vi "Drive Controller.vi"(8 "error in":errorcluster) -> ()   [LabVIEW 2019]
doc: "This VI executes continuously carrying out the current operation and responding to updates or new operation requests. It will often contain the timing or control code that is difficult to place directly in TeleOp. This VI generally opens all sensors and motors and isolates the rest of the robot code from knowing implementation details of how the operations are carried out."
uses:
  <vilib>/Rock Robotics/WPI/Framework/Completion Status.ctl
  Drive Setpoints.ctl
  Drive Operations.ctl
  <vilib>/Rock Robotics/WPI/ThirdParty/REV Robotics/SPARK MAX/Typedef/Spark MAX Control Type.ctl
panel:
  in  "Interactive Values":T1
  in  "Buttons":cluster{"Execute Cmd":bool, "Abort Cmd":bool}
  out "Command Timing":cluster{"Start Time (ms)":u32, "Iterations":i32}
  out "Status":T3
  out "Current\nCmd":string
  # "Tip: The graph shows the motor setpoints. It may also be helpful to observe inputs and sensor values.\nYou may also want to display tuning or debugging controls."
  # "Interactive Command: You may fill in the settings for a command\nand schedule it with the Execute button. You can observe and abort\nany command while fine tuning the code for the controller."
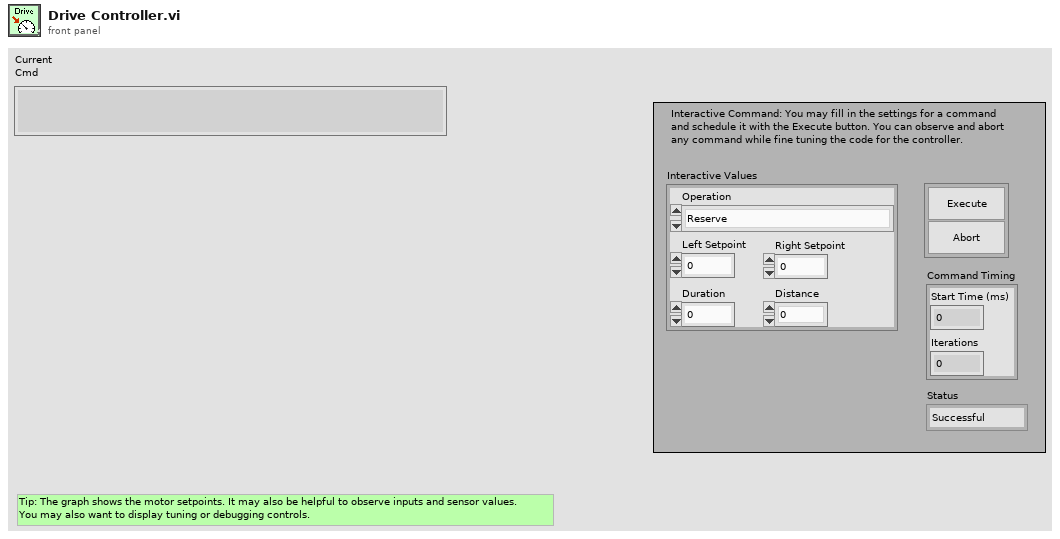
[diagram p1: front panel]
types:
  T1 = typedef "Drive Setpoints.ctl" = cluster{"Operation":T2, "Left Setpoint":dbl, "Right Setpoint":dbl, "Duration":dbl, "Distance":dbl}
  T2 = typedef "Drive Operations.ctl" = enum16{"Reserve", "Read Current", "Immediate", "Drive for Time", "Drive for Distance"}
  T3 = typedef "Completion Status.ctl" = enum16{"Successful", "Aborted", "Incomplete"}
  T4 = typedef "WPI_MotorControlDeviceRef.ctl" = cluster{"DeviceStatus":errorcluster, "Type":T5, "PWM":cluster{"PWM Channel":T6, "DeadBand":T7}, "CAN":cluster{"Device Number":u8, "SetOutput VI Ref":variant, "GetOutput VI Ref":variant, "Enable VI Ref":variant, "Disable VI Ref":variant, "Data":variant}, "Invert":bool, "DIO PWM":cluster{"PWM \"Enable\" Channel":T6, "DIOChannel":T8, "PWM Rate":dbl}}
  T5 = typedef "WPI_MotorControlType.ctl" = enum16{"PWM", "CAN", "DIO PWM"}
  T6 = typedef "FPGA_DIOPWMChannel.ctl" = enum8{"PWM 0", "PWM 1", "PWM 2", "PWM 3", "PWM 4", "PWM 5", "PWM 6", "PWM 7", "PWM 8", "PWM 9", "PWM MXP 0", "PWM MXP 1", "PWM MXP 2", "PWM MXP 3", "PWM MXP 4", "PWM MXP 5", "PWM MXP 6", "PWM MXP 7", "PWM MXP 8", "PWM MXP 9", "Invalid"}
  T7 = typedef "WPI_PWMDeadband.ctl" = cluster{"Name":string, "maxPositivePwm":i32, "minPositivePwm":i32, "centerPwm":i32, "maxNegativePwm":i32, "minNegativePwm":i32, "angularRange":u16}
  T8 = typedef "FPGA_DIOChannel.ctl" = enum8{"DIO 0", "DIO 1", "DIO 2", "DIO 3", "DIO 4", "DIO 5", "DIO 6", "DIO 7", "DIO 8", "DIO 9", "DIO MXP 0", "DIO MXP 1", "DIO MXP 2", "DIO MXP 3", "DIO MXP 4", "DIO MXP 5", "DIO MXP 6", "DIO MXP 7", "DIO MXP 8", "DIO MXP 9", "DIO MXP 10", "DIO MXP 11", "DIO MXP 12", "DIO MXP 13", "DIO MXP 14", "DIO MXP 15", "SPI Port CS1", "SPI Port CS2", "SPI Port CS3", "SPI Port MISO", "SPI Port MOSI", "Invalid"}
  T9 = typedef "Command Status Info.ctl" = cluster{"Name":string, "Status":T3, "notifier out":T10}
  T10 = typedef "Completion Notifier.ctl" = refnum<notifier>
  T11 = cluster{"SubSystem Data":T1, cluster{"Start Time (ms)":u32, "Iterations":i32}, cluster{"Command Info":T9, "Description":string, "Default Command":T1, "queue out":refnum<queue>, "Subsystem Name":string}}
  T12 = typedef "Spark MAX Control Type.ctl" = enum16{"Percent VBus", "Voltage", "Velocity", "Position", "Smart Motion", "Current", "Smart Velocity"}
  T13 = cluster{"SubSystem Data":T1, cluster{"Start Time (ms)":u32, "Iterations":i32}, "Default Command Arguments":cluster{"Command Info":T9, "Description":string, "Default Command":T1, "queue out":refnum<queue>, "Subsystem Name":string}}
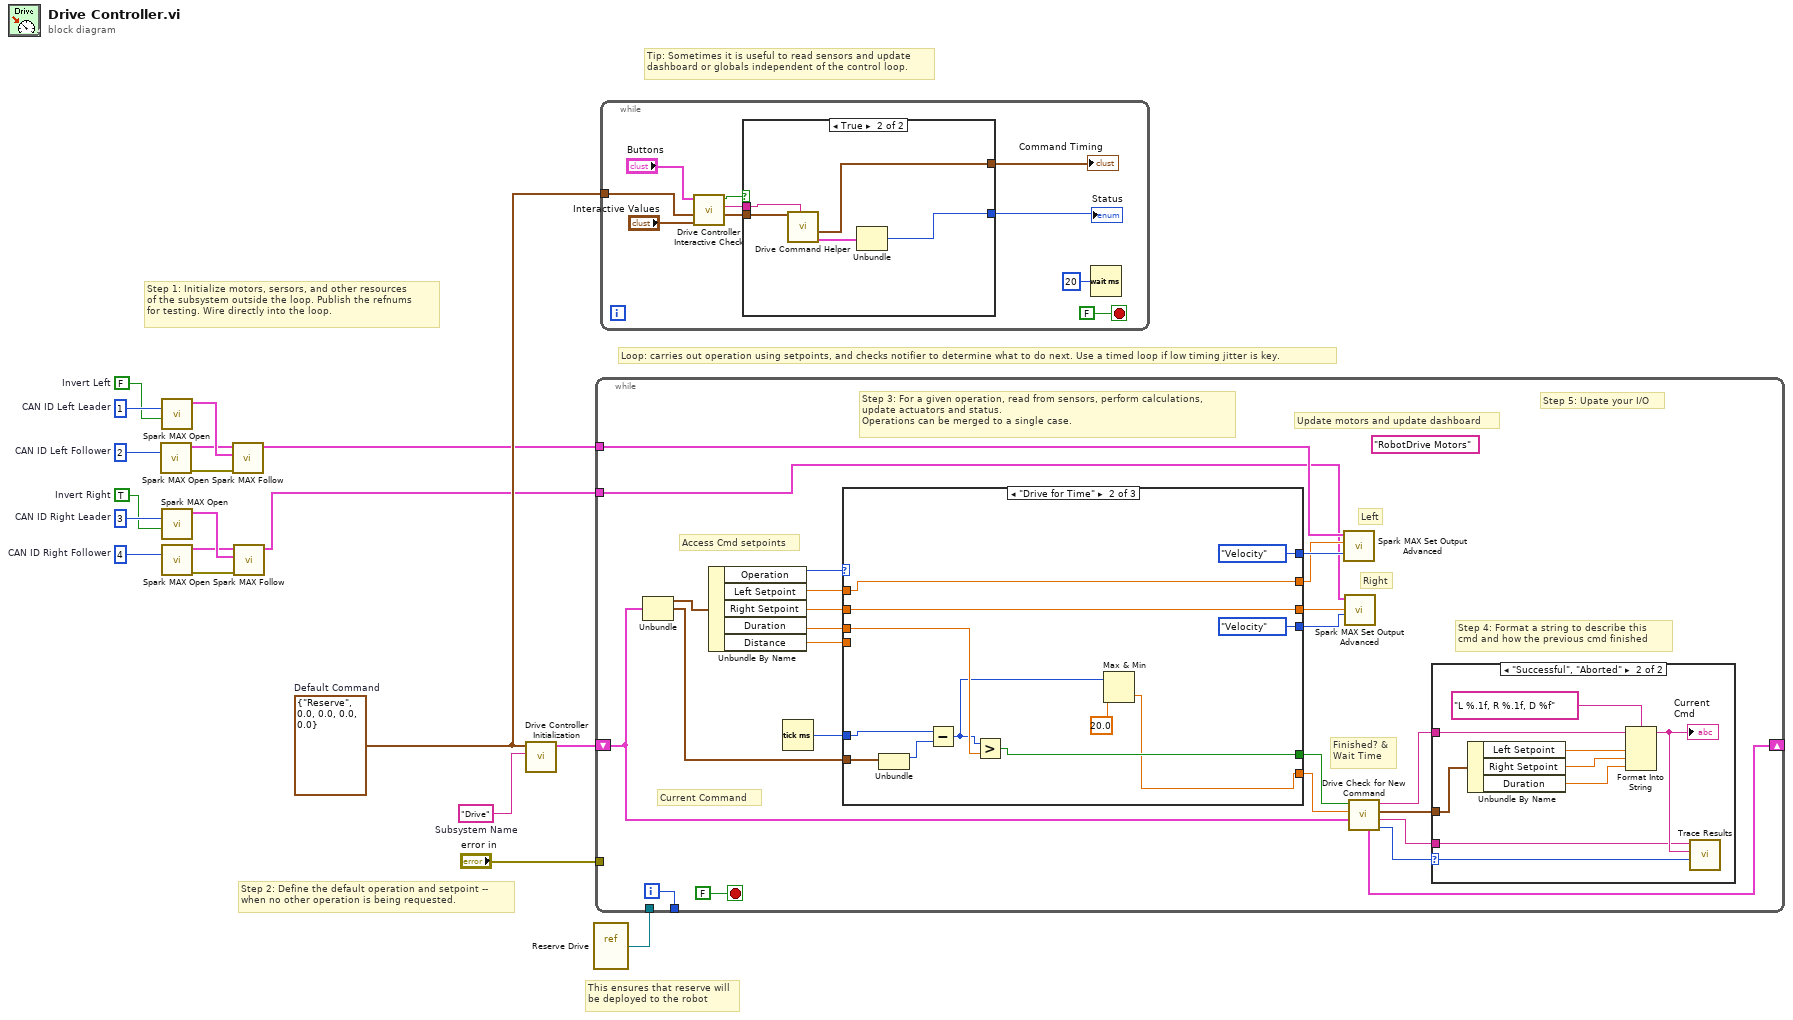
[diagram p0: block diagram]
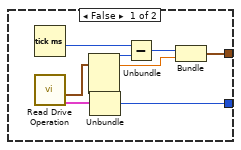
[diagram p2: hidden frame]
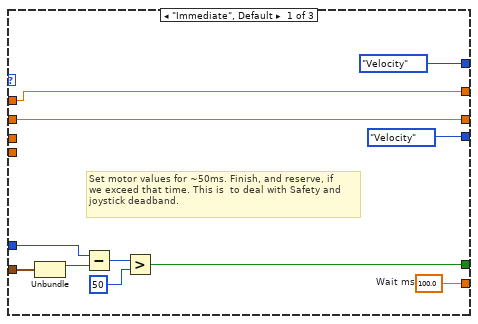
[diagram p4: hidden frame]
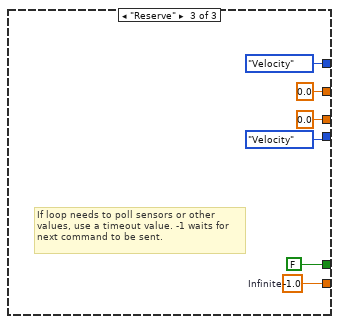
[diagram p5: hidden frame]
diagram:
  w3 = FALSE  # Invert Left
  w4 = TRUE  # Invert Right
  w6 = u8 3  # CAN ID Right Leader
  w5 = u8 4  # CAN ID Right Follower
  w12 = u8 1  # CAN ID Left Leader
  w13 = u8 2  # CAN ID Left Follower
  w15 = T1 {"Operation"=enum."Reserve", "Left Setpoint"=0.0, "Right Setpoint"=0.0, "Duration"=0.0, "Distance"=0.0}  # Default Command
  w19 = "Drive"  # Subsystem Name
  # "This ensures that reserve will\nbe deployed to the robot"
  # "Tip: Sometimes it is useful to read sensors and update\ndashboard or globals independent of the control loop."
  # "Step 2: Define the default operation and setpoint --\nwhen no other operation is being requested."
  # "Step 1: Initialize motors, sersors, and other resources\nof the subsystem outside the loop. Publish the refnums\nfor testing. Wire directly into the loop."
  # "Loop: carries out operation using setpoints, and checks notifier to determine what to do next. Use a timed loop if low timing jitter is key."
  n1 = call <vilib>:"Spark MAX Open.vi"("Device Number"=w13) -> ("error out"=w9:errorcluster, "MotorControlDeviceRef"=w10:T4)  [unwired: 9 in]
  n2 = call <vilib>:"Spark MAX Open.vi"("Invert"=w3, "Device Number"=w12) -> ("MotorControlDeviceRef"=w11:T4)  [unwired: 8 in, 1 out]
  n3 = call <vilib>:"Spark MAX Open.vi"("Invert"=w4, "Device Number"=w6) -> ("MotorControlDeviceRef"=w14:T4)  [unwired: 8 in, 1 out]
  n4 = call <vilib>:"Spark MAX Open.vi"("Device Number"=w5) -> ("error out"=w8:errorcluster, "MotorControlDeviceRef"=w7:T4)  [unwired: 9 in]
  n5 = call <vilib>:"Spark MAX Follow.vi"("error in (no error)"=w9, "Master Controller"=w11, "MotorControlDeviceRef"=w10) -> ("MotorControlDeviceRef"=w1:T4)  [unwired: 7 in, 1 out]
  n6 = call <vilib>:"Spark MAX Follow.vi"("error in (no error)"=w8, "Master Controller"=w14, "MotorControlDeviceRef"=w7) -> ("MotorControlDeviceRef"=w2:T4)  [unwired: 7 in, 1 out]
  n7 = call "Drive Controller Initialization.vi"("Subsystem Name"=w19, "Default Command"=w15) -> ("Current Command"=w17:T11)  [unwired: 9 in]
  n8 = vi-ref "Reserve Drive.vi"() -> (w16:refnum<vi>)
  n9 = while {
    shift-right: [w34] -> _
    shift-left: w17 -> [w27]
    tunnel: [w42] -> _
    tunnel: "error in" -> [_]
    tunnel: w16 -> [_]
    tunnel: w2 -> [w21]
    tunnel: w1 -> [w22]
    i -> [w42]
    stop <- FALSE stop-if-true
    (unwired) "RobotDrive Motors" ("Name")
    # "Left"
    # "Right"
    # "Step 5: Upate your I/O"
    # "Step 4: Format a string to describe this\ncmd and how the previous cmd finished"
    # "Current Command"
    # "Update motors and update dashboard"
    # "Access Cmd setpoints"
    # "Finished? &\nWait Time"
    # "Step 3: For a given operation, read from sensors, perform calculations,\nupdate actuators and status.\nOperations can be merged to a single case."
    n10 = Unbundle(w27) -> ("SubSystem Data"=w41:T1, w28:cluster{"Start Time (ms)":u32, "Iterations":i32})  [unwired: 1 out]
    n11 = Unbundle By Name(w41) -> ("Operation"=w40:T2, "Left Setpoint"=w39:dbl, "Right Setpoint"=w38:dbl, "Duration"=w37:dbl, "Distance"=w20:dbl)
    n12 = Tick Count (ms)() -> (millisecond timer value=w36:u32)
    n13 = case shown="\"Drive for Time\"" w40 {
      tunnel: [w63 w65 w81] -> w33
      tunnel: [w58 w68 FALSE ("ignore previous (F)")] -> w32
      tunnel: w28 -> [w57 w73 _]
      tunnel: w39 -> [w56 w70 _]
      tunnel: w38 -> [w55 w69 _]
      tunnel: w37 -> [_ w67 _]
      tunnel: w36 -> [w59 w71 _]
      tunnel: [w56 w70 0.0 ("Left Setpoint")] -> w24
      tunnel: [w55 w69 0.0 ("Right Setpoint")] -> w23
      tunnel: [Spark_MAX_Control_Type."Velocity" ("Control Mode") Spark_MAX_Control_Type."Velocity" ("Control Mode") Spark_MAX_Control_Type."Velocity" ("Control Mode")] -> w26
      tunnel: [Spark_MAX_Control_Type."Velocity" ("Control Mode") Spark_MAX_Control_Type."Velocity" ("Control Mode") Spark_MAX_Control_Type."Velocity" ("Control Mode")] -> w25
      tunnel: w20 -> [_ _ _]
      frame "Immediate", Default {
        w63 = 100.0  # Wait ms
        # "Set motor values for ~50ms. Finish, and reserve, if\nwe exceed that time. This is  to deal with Safety and\njoystick deadband."
        n14 = Unbundle(w57) -> ("Start Time (ms)"=w60:u32)  [unwired: 1 out]
        n15 = Subtract(x=w59, y=w60) -> (x-y=w61:u32)
        n16 = Greater?(x=w61, y=u8 50 ("Left Motor")) -> (0:w58:bool)
      }
      frame "Drive for Time" {
        n17 = Unbundle(w73) -> ("Start Time (ms)"=w72:u32)  [unwired: 1 out]
        n18 = Subtract(x=w71, y=w72) -> (x-y=w64:u32)
        n19 = Greater?(x=w64, y=w67) -> (0:w68:bool)
        n20 = Max & Min(x=w64, y=20.0) -> (min(x,y)=w65:dbl)  [unwired: 1 out]
      }
      frame "Reserve" {
        w81 = -1.0  # Infinite
        # "If loop needs to poll sensors or other\nvalues, use a timeout value. -1 waits for\nnext command to be sent."
      }
    }
    n21 = call <vilib>:"Spark MAX Set Output Advanced.vi"("Control Mode"=w25, "Setpoint"=w24, "MotorControlDevRef"=w22) -> ()  [unwired: 7 in, 2 out]
    n22 = call <vilib>:"Spark MAX Set Output Advanced.vi"("Control Mode"=w26, "Setpoint"=w23, "MotorControlDevRef"=w21) -> ()  [unwired: 7 in, 2 out]
    n23 = call "Drive Check for New Command.vi"("input cluster"=w27, "Wait time (ms)"=w33, "Finished?"=w32) -> ("Completion"=w35:T3, "Subsystem Name"=w29:string, "Current Command"=w30:T1, "Initial Trace String"=w31:string, "Next Command"=w34:T13)  [unwired: 4 in]
    n24 = case shown="\"Successful\", \"Aborted\"" w35 {
      selector: w35 -> [_ w52]
      tunnel: w31 -> [_ w47]
      tunnel: w30 -> [_ w48]
      tunnel: w29 -> [_ w44]
      frame "Incomplete", Default {
        # "Continuing current command"
      }
      frame "Successful", "Aborted" {
        # "Report and setup for next command"
        n25 = Unbundle By Name(w48) -> ("Left Setpoint"=w50:dbl, "Right Setpoint"=w51:dbl, "Duration"=w45:dbl)
        n26 = Format Into String(format string="L %.1f, R %.1f, D %f", initial string=w47, w50, w51, w45) -> (resulting string=w46:string)  [unwired: 1 in, 1 out]
        "Current\nCmd" <- w46
        n27 = call <vilib>:"Trace Results.vi"("Status of previous command"=w52, "Description"=w46, "Subsystem"=w44) -> ()  [unwired: 9 in]
      }
    }
  }
  n28 = while {
    tunnel: w15 -> [w83]
    stop <- FALSE stop-if-true
    n29 = call "Drive Controller Interactive Check.vi"("Interactive Command In"="Interactive Values", "Default Command"=w83, "Buttons"="Buttons") -> ("Interactive Command Out"=w85:T1, "Trace String"=w86:string, "Schedule"=w87:bool)  [unwired: 6 in]
    n30 = case shown="True" w87 {
      tunnel: [w96 w104] -> w88
      tunnel: [w95 w100] -> w89
      tunnel: w86 -> [_ w102]
      tunnel: w85 -> [_ w101]
      frame False {
        n31 = Tick Count (ms)() -> (millisecond timer value=w99:u32)
        n32 = call "Read Drive Operation.vi"() -> ("Command Info"=w93:T9, "SubSystem Data"=w92:T1)  [unwired: 9 in, 1 out]
        n33 = Unbundle(w92) -> ("Operation"=w97:T2, "Left Setpoint"=w94:dbl)  [unwired: 3 out]
        n34 = Unbundle(w93) -> ("Status"=w96:T3)  [unwired: 2 out]
        n35 = Subtract(x=w99, y=w97) -> (x-y=w98:u32)
        n36 = Bundle(w98, "Left Setpoint"=w94) -> (w95:cluster{u32, "Left Setpoint":dbl})  [unwired: 1 in]
      }
      frame True {
        n37 = call "Drive Command Helper.vi"("Description"=w102, "SubSystem Data"=w101) -> ("Command Info Out"=w103:T9, "Command Timing"=w100:cluster{"Start Time (ms)":u32, "Iterations":i32})  [unwired: 7 in, 1 out]
        n38 = Unbundle(w103) -> ("Status"=w104:T3)  [unwired: 2 out]
      }
    }
    "Status" <- w88
    "Command Timing" <- w89
    n39 = Wait (ms)(milliseconds to wait=u32 20) -> ()  [unwired: 1 out]
  }
